vi "Get Source Delay.vi"(8 "error in (no error)":errorcluster, 10 "Function (0: Volts)":u16(ring) items=["Volts", "Current"], 11 "VISA resource name":refnum<visa-resource-name>) -> (0 "error out":errorcluster, 2 "Source Delay":dbl, 3 "VISA resource name out":refnum<visa-resource-name>)   [LabVIEW 2020, in "Keithley 2450.lvlib"]
doc: "Gets source delay value for the selected source function."
uses:
  <instrlib>/Keithley 2450/Keithley 2450.lvlib
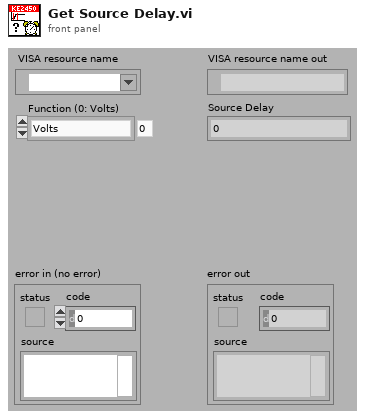
[diagram p1: front panel]
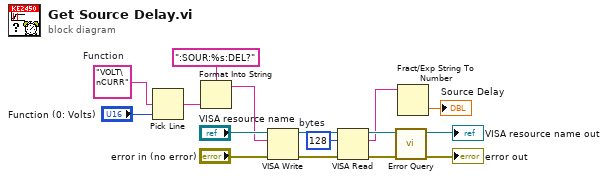
[diagram p0: block diagram]
diagram:
  w7 = u32 128  # bytes
  w10 = "VOLT\nCURR"  # Function
  n1 = Pick Line(multi-line string=w10, line index="Function (0: Volts)") -> (output string=w8:string)  [unwired: 1 out]
  n2 = Format Into String(format string=":SOUR:%s:DEL?", w8) -> (resulting string=w11:string)  [unwired: 2 in, 1 out]
  n3 = VISA Write(VISA resource name="VISA resource name", write buffer=w11, error in (no error)="error in (no error)") -> (VISA resource name out=w6:refnum<visa-resource-name>, error out=w4:errorcluster)  [unwired: 1 out]
  n4 = VISA Read(VISA resource name=w6, byte count=w7, error in (no error)=w4) -> (VISA resource name out=w5:refnum<visa-resource-name>, read buffer=w2:string, error out=w3:errorcluster)  [unwired: 1 out]
  n5 = call <instrlib>:"Error Query.vi"("error in (no error)"=w3, "VISA resource name"=w5) -> ("error out"=→"error out":errorcluster, "VISA resource name out"=→"VISA resource name out":refnum<visa-resource-name>)  [unwired: 8 out]
  n6 = Fract/Exp String To Number(string=w2) -> (number=→"Source Delay":dbl)  [unwired: 3 in, 1 out]
